vi "Read Lockin_Sweep.json.vi"(8 "error in (no error)":errorcluster, 10 "file (use dialog)":path, 11 "Transport in":refnum<class "Transport.lvclass">) -> (0 "error out":errorcluster, 2 "Sweep Configuration":T1 {"sweepTables"."Table" format="%#_3p"; "sweepTables"."Ch" min=1 max=16; "sweepChannels"."Table" format="%#_1f"; "sweepChannels"."Channel" min=1 max=128; "sweepChannels"."Start" format="%#_6p"; "sweepChannels"."End" format="%#_6p"}, 3 "Transport out":refnum<class "Transport.lvclass">)   [LabVIEW 2019, in "Transport.lvclass"]
uses:
  Transport.lvclass
  Typedefs/Lockin_Sweep JSON--Cluster.ctl
  <userlib>/LevyLab/Lockin-Multichannel/Instrument.DAQ/Typedefs/Sweep.Channel--Cluster--Array.ctl
  <userlib>/LevyLab/Lockin-Multichannel/Instrument.DAQ/Typedefs/Sweep.Channel--Cluster.ctl
  <userlib>/LevyLab/Lockin-Multichannel/Instrument.DAQ/Typedefs/Sweep.Pattern--Enum.ctl
  011176b6-c653-49bb-be18-96c3656e62d6.vi
  <vilib>/JDP Science/JSONtext/JSON text to Variant.vi
  <vilib>/JDP Science/JSONtext/LVClass Serializer/JSONtext LVClass Serializer.lvclass
  <userlib>/LevyLab/Lockin-Multichannel/Instrument.DAQ/Instrument.DAQ.lvclass
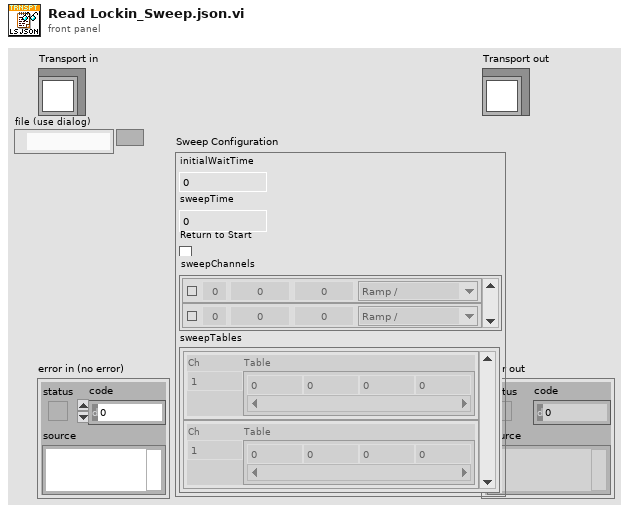
[diagram p1: front panel]
types:
  T1 = typedef "Transport.lvclass/Lockin_Sweep JSON--Cluster.ctl" = cluster{"initialWaitTime":dbl, "sweepTime":dbl, "Return to Start":bool, "sweepChannels":T2, "sweepTables":cluster{"Ch":i32, "Table":dbl[]}[]}
  T2 = typedef "Instrument.Lockin.lvlib/Instrument.DAQ.lvclass/Sweep.Channel--Cluster--Array.ctl" = T3[]
  T3 = typedef "Instrument.Lockin.lvlib/Instrument.DAQ.lvclass/Sweep.Channel--Cluster.ctl" = cluster{"Enable?":bool, "Channel":u16, "Start":dbl, "End":dbl, "Pattern":T4, "Table":dbl[]}
  T4 = typedef "Instrument.Lockin.lvlib/Instrument.DAQ.lvclass/Sweep.Pattern--Enum.ctl" = enum16{"Ramp /", "Ramp /\\", "Smooth Ramp _/", "Smooth Ramp _/\\_", "Table"}
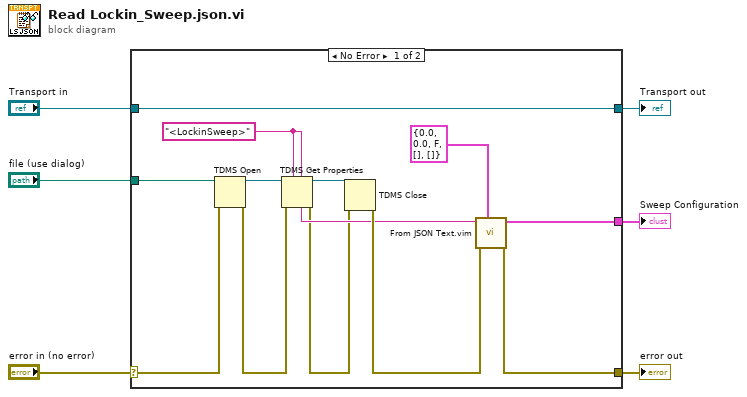
[diagram p0: block diagram]
diagram:
  n1 = case shown="No Error" "error in (no error)" {
    selector: "error in (no error)" -> [w17 w21]
    tunnel: [w14 w21] -> w5
    tunnel: [w19 w20] -> w3
    tunnel: "Transport in" -> [w19 w20]
    tunnel: [w16 _] -> w2
    tunnel: "file (use dialog)" -> [w18 _]
    frame No Error {
      w13 = "<LockinSweep>" ("group name")
      n2 = TDMS Open(8:w17, 11:w18) -> (0:w11:errorcluster, 3:w12:refnum<k34>)  [unwired: 5 in]
      n3 = TDMS Get Properties(5:w13, 7:w13, 8:w11, 11:w12) -> (0:w8:errorcluster, 3:w10:refnum<k34>, 4:w9:string)  [unwired: 2 in, 3 out]
      n4 = TDMS Close(8:w8, 11:w10) -> (0:w15:errorcluster)  [unwired: 1 out]
      n5 = call "From JSON Text.vim"("Data Type and Default Value"=T1 {"initialWaitTime"=0.0, "sweepTime"=0.0, "Return to Start"=FALSE, "sweepChannels"=[], "sweepTables"=[]} ("Lockin_Sweep"), "error in (no error)"=w15, "JSON"=w9) -> ("error out"=w14:errorcluster, "Data out"=w16:T1)  [unwired: 7 in]
    }
    frame Error {
    }
  }
  "error out" <- w5
  "Transport out" <- w3
  "Sweep Configuration" <- w2
